vi "Chi-Squared PDF.vi"(10 "k":i32=1, 11 "x":dbl=1.0) -> (0 "error":i32, 3 "pdf(x)":dbl=0.24197072451914334)   [LabVIEW 2020, in "NI_Gmath.lvlib"]
doc: "Computes the continuous probability density function (PDF) of various distributions. You must manually select the polymorphic instance to use."
uses:
  NI_Gmath.lvlib
  st_error_code.ctl
panel:
  # "Chi-Squared PDF"
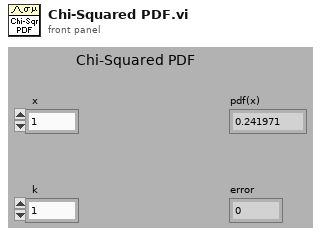
[diagram p1: front panel]
types:
  T1 = typedef "NI_Gmath.lvlib/st_error_code.ctl" = i32
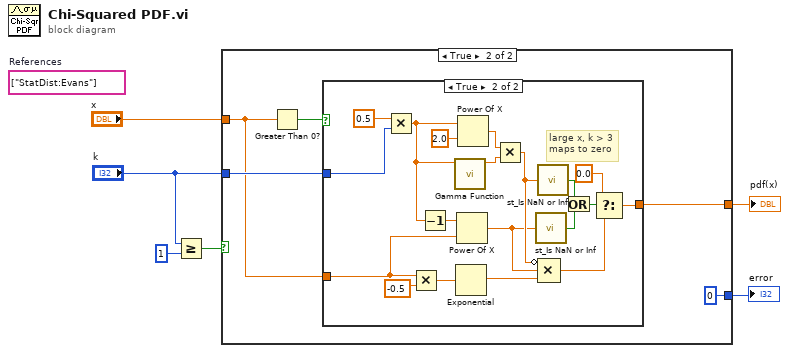
[diagram p0: block diagram]
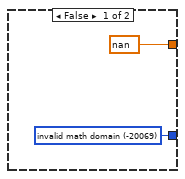
[diagram p2: hidden frame]
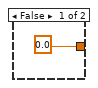
[diagram p3: hidden frame]
diagram:
  (unwired) string[] ["StatDist:Evans"]  # References
  n1 = Greater Or Equal?(x="k", y=1) -> (x >= y?=w1:bool)
  n2 = case shown="True" w1 {
    tunnel: [w7 0 ("invalid math domain")] -> w6
    tunnel: [nan w12] -> w5
    tunnel: "x" -> [_ w10]
    tunnel: "k" -> [_ w11]
    frame False {
      w7 = T1 -20069 items=["invalid math domain"=-20069, "Fourier interpolation size m >= n"=-20070, "empty array"=-20003] ("stat interp error code")
    }
    frame True {
      n3 = Greater Than 0?(x=w10) -> (x > 0?=w9:bool)
      n4 = case shown="True" w9 {
        tunnel: [0.0 w20] -> w12
        tunnel: w10 -> [_ w28]
        tunnel: w11 -> [_ w32]
        frame False {
        }
        frame True {
          # "large x, k > 3\nmaps to zero"
          n5 = Multiply(x=0.5, y=w32) -> (x*y=w30:dbl)
          n6 = Multiply(x=w28, y=-0.5 ("x")) -> (x*y=w26:dbl)
          n7 = Decrement(x=w30) -> (x-1=w29:dbl)
          n8 = call "Gamma Function.vi"("x"=w30) -> ("g(x)"=w19:dbl)  [unwired: 10 in]
          n9 = Exponential(1:w26) -> (0:w17:dbl)
          n10 = Power Of X(1:w28, 2:w29) -> (0:w16:dbl)
          n11 = Power Of X(1:2.0 ("x"), 2:w30) -> (0:w25:dbl)
          n12 = Multiply(x=w25, y=w19) -> (x*y=w18:dbl)
          n13 = call "st_Is NaN or Inf.vi"("x"=w16) -> ("isNaN(x) || isInf(x)"=w22:bool)  [unwired: 4 in]
          n14 = call "st_Is NaN or Inf.vi"("x"=w18) -> ("isNaN(x) || isInf(x)"=w23:bool)  [unwired: 4 in]
          n15 = Compound Arithmetic op=MULTIPLY(invert w18, w16, w17) -> (w15:dbl)
          n16 = Or(x=w23, y=w22) -> (x .or. y?=w24:bool)
          n17 = Select(t=0.0, s=w24, f=w15) -> (s? t:f=w20:dbl)
        }
      }
    }
  }
  "pdf(x)" <- w5
  "error" <- w6
